vi "MINST_pattern_1D_to_2DX_Y.vi"(3 "pattern 1D":i32[](array[numeric])) -> (0 "Pattern_Y":i16=9, 1 "2D(28_28)":i32[][](array[numeric]))   [LabVIEW 2021]
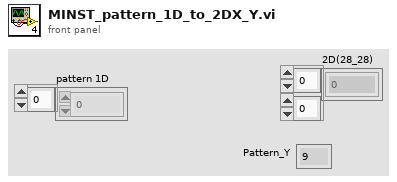
[diagram p1: front panel]
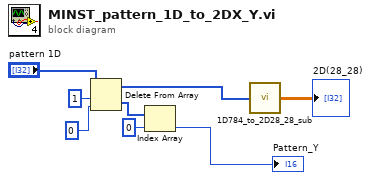
[diagram p0: block diagram]
diagram:
  n1 = Delete From Array(array="pattern 1D", length=1, index=0) -> (deleted portion=w6:i32[], array with subset deleted=w2:i32[])
  n2 = Index Array(array=w6, index=0) -> (element=→"Pattern_Y":i32)
  n3 = call "1D784_to_2D28_28_sub.vi"("1D(784)"=w2) -> ("2D(28_28)"=→"2D(28_28)":dbl[][])
